vi "Task Type.vi"(11 "SimTask in":refnum<class "SimTask.lvclass">) -> (2 "Task Type":string)   [LabVIEW 2020, in "VolatusDemo.lvlib" / "SimTask.lvclass"]
uses:
  SimTask.lvclass
  SimTask.lvclass/SimTask.ctl
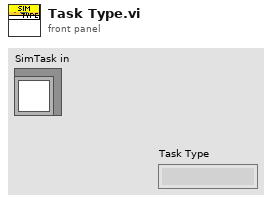
[diagram p1: front panel]
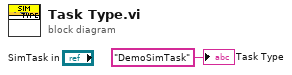
[diagram p0: block diagram]
diagram:
  "Task Type" <- "DemoSimTask" ("Task Type")
